vi "MCCPMTupdate.vi"(0 "MCCPMT in":refnum<class "MCCPMT.lvclass">, 5 "pmt voltage 1":dbl, 7 "pmt voltage 2":dbl, 9 "pmt voltage 3":dbl, 11 "error in (no error)":errorcluster) -> (4 "MCCPMT out":refnum<class "MCCPMT.lvclass">, 15 "error out":errorcluster)   [LabVIEW 2012, in "MCCPMT.lvclass"]
uses:
  MCCPMT.lvclass
  MCCPMT.lvclass/MCCPMT.ctl
  <vilib>/ULx/Create Channel.llb/ULx Create Channel (AO-Voltage-Basic).vi
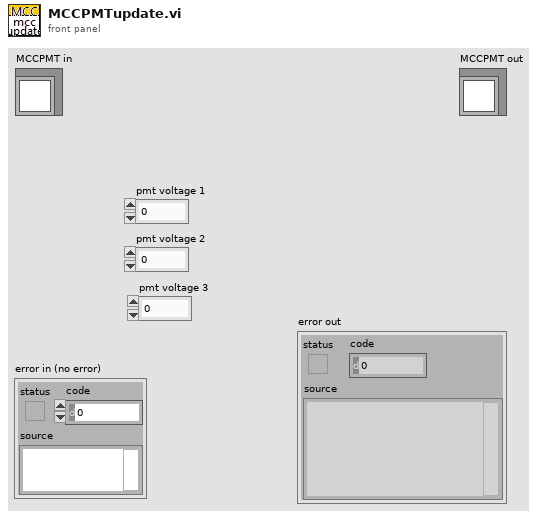
[diagram p1: front panel]
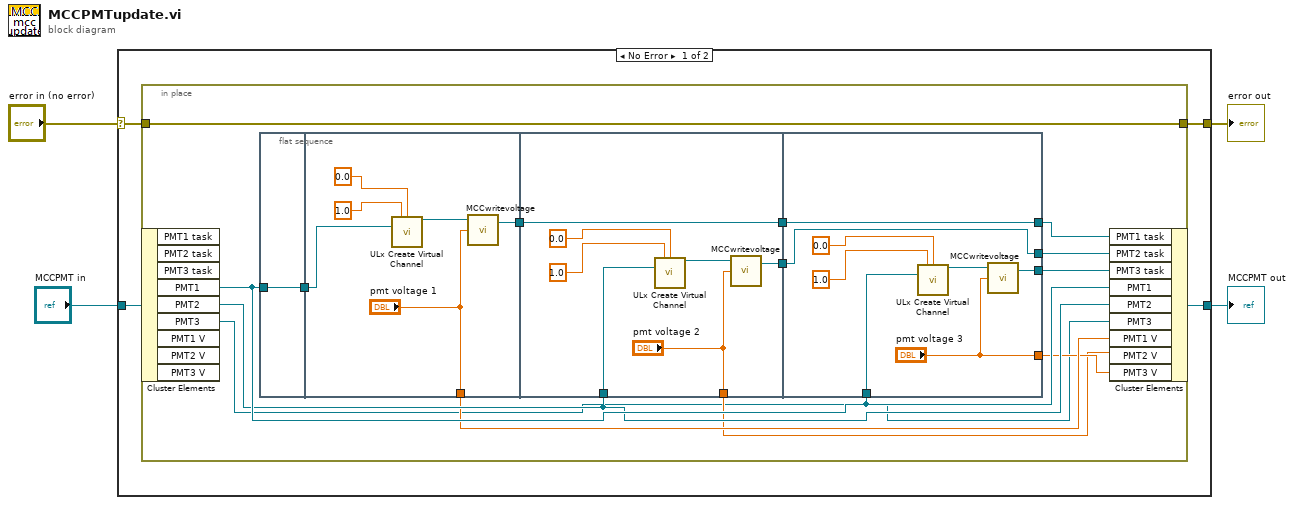
[diagram p0: block diagram]
diagram:
  n1 = case shown="No Error" "error in (no error)" {
    selector: "error in (no error)" -> [w6 w46]
    tunnel: [w5 w46] -> w3
    tunnel: [w7 w45] -> w1
    tunnel: "MCCPMT in" -> [w8 w45]
    frame No Error {
      n2 = in-place {
        in-place-border: w6 -> [w22]
        in-place-border: [w22] -> w5
        n3 = in-place-cluster #1(w8) -> ("PMT1"=w21:refnum<k21>, "PMT2"=w19:refnum<k21>, "PMT3"=w9:refnum<k21>)  [unwired: 6 out]
        n4 = flat-sequence {
          tunnel: w21 -> [w23]
          tunnel: [w23] -> w16
          tunnel: [w25] -> w20
          tunnel: w16 -> [w28]
          tunnel: ["pmt voltage 1"] -> w15
          tunnel: w20 -> [w36]
          tunnel: w19 -> [w33]
          tunnel: [w36] -> w14
          tunnel: [w31] -> w13
          tunnel: ["pmt voltage 2"] -> w10
          tunnel: [w43] -> w17
          tunnel: [w44] -> w18
          tunnel: w14 -> [w44]
          tunnel: w13 -> [w43]
          tunnel: [w39] -> w12
          tunnel: ["pmt voltage 3"] -> w11
          tunnel: w9 -> [w37]
          frame #0 {
          }
          frame #1 {
            n5 = call-poly <vilib>:"ULx Create Virtual Channel.vi"("maximum value"=1.0, "minimum value"=0.0, "physical channels"=w28) -> ("task out"=w29:refnum<k24>)  [unwired: 11 in, 1 out]
            n6 = call "MCCwritevoltage.vi"("output voltage"="pmt voltage 1", "task in"=w29) -> ("task out"=w25:refnum<k24>)  [unwired: 1 in, 1 out]
          }
          frame #2 {
            n7 = call-poly <vilib>:"ULx Create Virtual Channel.vi"("maximum value"=1.0, "minimum value"=0.0, "physical channels"=w33) -> ("task out"=w32:refnum<k24>)  [unwired: 11 in, 1 out]
            n8 = call "MCCwritevoltage.vi"("output voltage"="pmt voltage 2", "task in"=w32) -> ("task out"=w31:refnum<k24>)  [unwired: 1 in, 1 out]
          }
          frame #3 {
            n9 = call-poly <vilib>:"ULx Create Virtual Channel.vi"("maximum value"=1.0, "minimum value"=0.0, "physical channels"=w37) -> ("task out"=w40:refnum<k24>)  [unwired: 11 in, 1 out]
            n10 = call "MCCwritevoltage.vi"("output voltage"="pmt voltage 3", "task in"=w40) -> ("task out"=w39:refnum<k24>)  [unwired: 1 in, 1 out]
          }
        }
        n11 = in-place-cluster #1("PMT1 task"=w18, "PMT2 task"=w17, "PMT3 task"=w12, "PMT1"=w21, "PMT2"=w19, "PMT3"=w9, "PMT1 V"=w15, "PMT2 V"=w10, "PMT3 V"=w11) -> (w7:refnum<class "MCCPMT.lvclass">)
      }
    }
    frame Error {
    }
  }
  "error out" <- w3
  "MCCPMT out" <- w1
